vi "StartMicron.vi"(7 "Alias Name":string, 8 "error in":errorcluster, 9 "Other Args":string, 10 "Port":i32, 11 "Micron Path":path) -> (0 "error out":errorcluster, 3 "Connection String":string)   [LabVIEW 2019, in "MicronHelper.lvlib"]
uses:
  MicronHelper.lvlib
  <vilib>/SLL Toolkit/SLL File IO/SLL File IO.lvlib
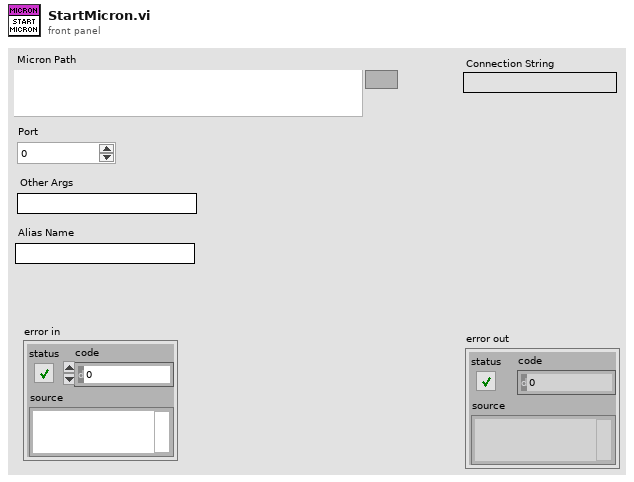
[diagram p1: front panel]
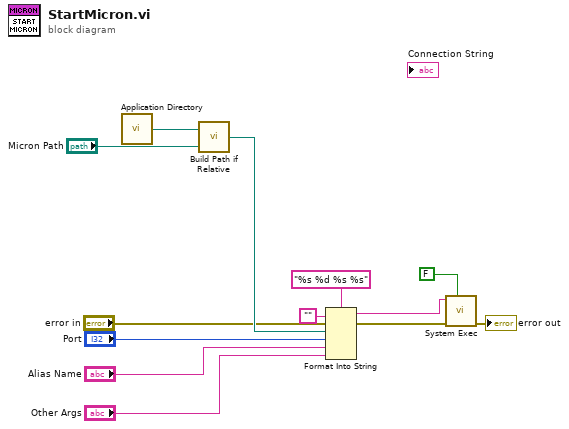
[diagram p0: block diagram]
diagram:
  n1 = call <vilib>:"Application Directory.vi"() -> ("Application Directory"=w8:path)
  n2 = call <vilib>:"Build Path if Relative.vi"("Relative or Absolute Path"="Micron Path", "Base Path"=w8) -> ("Path Out"=w7:path)
  n3 = Format Into String(format string="%s %d %s %s", initial string="", error in="error in", w7, "Port", "Alias Name", "Other Args") -> (resulting string=w9:string, error out=w12:errorcluster)
  n4 = call <vilib>:"System Exec.vi"("wait until completion? (T)"=FALSE, "error in (no error)"=w12, "command line"=w9) -> ("error out"=→"error out":errorcluster)  [unwired: 5 in, 3 out]
